vi "formula node exercise.vi"() -> ()   [LabVIEW 2018]
panel:
  out "Waveform Graph":dbl[](graph)
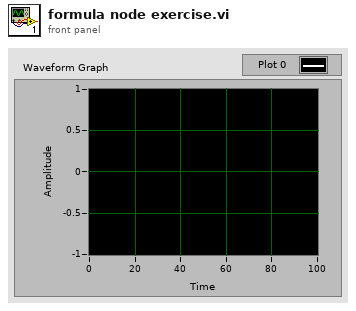
[diagram p1: front panel]
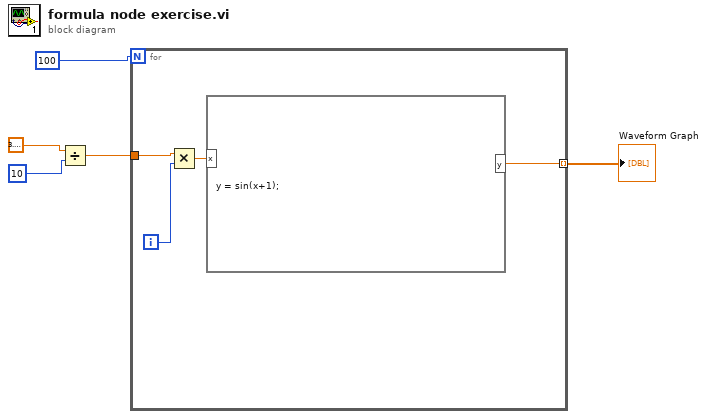
[diagram p0: block diagram]
diagram:
  n1 = Divide(x=3.141592653589793, y=10) -> (x/y=w4:dbl)
  n2 = for {
    N: 100 -> [_]
    tunnel: [w7] -> w1 mode=indexing
    tunnel: w4 -> [w6]
    i -> [w8]
    n3 = Multiply(x=w6, y=w8) -> (x*y=w9:dbl)
    n4 = formula code="y = sin(x+1);"("x"=w9) -> ("y"=w7:dbl)
  }
  "Waveform Graph" <- w1
